vi "Default Instrument Setup.vi"(8 "error in (no error)":errorcluster, 11 "VISA resource name":refnum<visa-resource-name>) -> (0 "error out":errorcluster, 3 "VISA resource name out":refnum<visa-resource-name>)   [LabVIEW 2019, in "Keithley 6517.lvlib"]
doc: "Sends a default command string to the instrument whenever a new VISA session is opened, or the instrument is reset. Use this VI as a subVI for the <b>Initialize</b> and <b>Reset</b> VIs. Altering this VI could cause these two VIs to operate incorrectly."
uses:
  Keithley 6517.lvlib
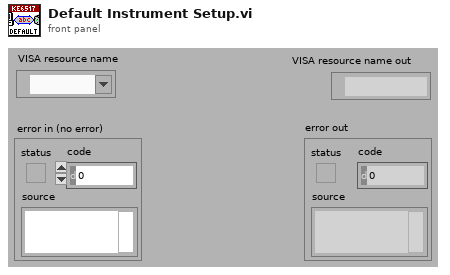
[diagram p1: front panel]
types:
  T1 = typedef "Keithley 6517.lvlib/Extended User Data.ctl" = cluster{"Instrument Model":i32}
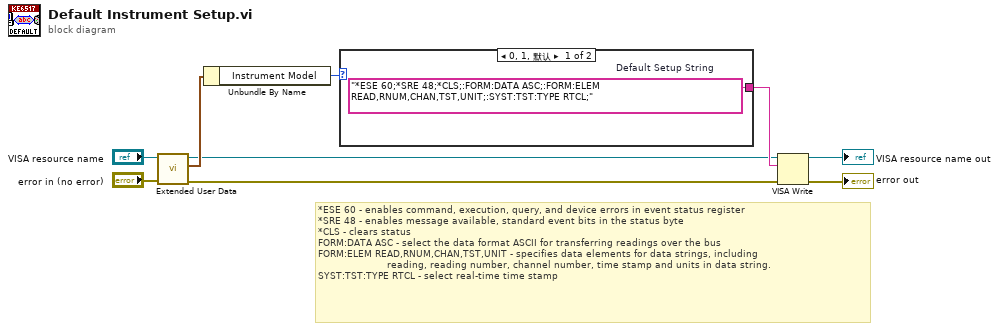
[diagram p0: block diagram]
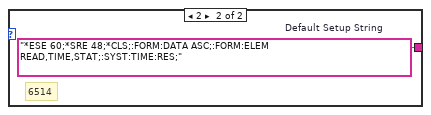
[diagram p2: hidden frame]
diagram:
  # "*ESE 60 - enables command, execution, query, and device errors in event status register\n*SRE 48 - enables message available, standard event bits in the status byte\n*CLS - clears status\nFORM:DATA ASC - select the data format ASCII for transferring readings over the bus \nFORM:ELEM READ,RNUM,CHAN,TST,UNIT - specifies data elements for data strings, including \n                       reading, reading number, channel number, time stamp and units in data string.\nSYST:TST:TYPE RTCL - select real-time time stamp"
  n1 = call "Extended User Data.vi"("error in (no error)"="error in (no error)", "VISA resource name"="VISA resource name") -> ("error out"=w2:errorcluster, "User Data Out"=w4:T1, "VISA resource name out"=w1:refnum<visa-resource-name>)  [unwired: 7 in]
  n2 = Unbundle By Name(w4) -> ("Instrument Model"=w3:i32)
  n3 = case shown="0, 1, 默认" w3 {
    tunnel: [w10 w11] -> w7
    frame 0, 1, Default {
      w10 = "*ESE 60;*SRE 48;*CLS;:FORM:DATA ASC;:FORM:ELEM READ,RNUM,CHAN,TST,UNIT;:SYST:TST:TYPE RTCL;"  # Default Setup String
    }
    frame 2 {
      w11 = "*ESE 60;*SRE 48;*CLS;:FORM:DATA ASC;:FORM:ELEM READ,TIME,STAT;:SYST:TIME:RES;"  # Default Setup String
      # "6514"
    }
  }
  n4 = VISA Write(VISA resource name=w1, write buffer=w7, error in (no error)=w2) -> (VISA resource name out=→"VISA resource name out":refnum<visa-resource-name>, error out=→"error out":errorcluster)  [unwired: 1 out]
